vi "Detect Framework From Application Domain.vi"(8 "error in (no error)":errorcluster) -> (0 "error out":errorcluster, 1 "Test Framework Instance":refnum<class "Test Framework.lvclass">, 2 "Test Framework Type":T1=enum."LVUnit")   [LabVIEW 2017, in "Framework.lvlib" / "Test Framework Factory.lvclass"]
uses:
  Test Framework Factory.lvclass
  Test Framework/Test Framework.lvclass
  Test Framework.ctl
  LVUnit Test Framework/LVUnit Test Framework.lvclass
  C:/Users/pasca/Projects/Home/lvunit/Framework/Test Framework/Test Framework.lvclass
  Framework.lvlib
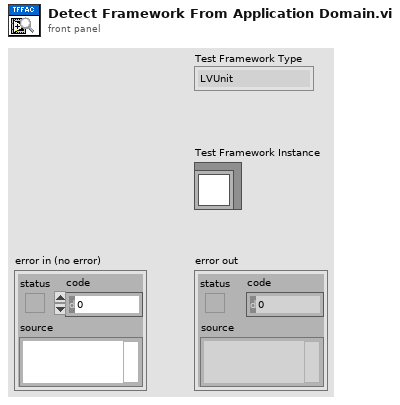
[diagram p1: front panel]
types:
  T1 = typedef "Framework.lvlib/Test Framework.ctl" = enum16{"Unknown", "LVUnit"}
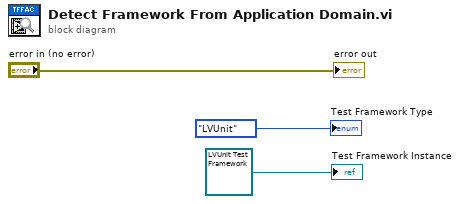
[diagram p0: block diagram]
diagram:
  "error out" <- "error in (no error)"
  "Test Framework Instance" <- refnum<class "LVUnit Test Framework.lvclass"> refnum ("Framework.lvlib:LVUnit Test Framework.lvclass")
  "Test Framework Type" <- Test_Framework."LVUnit" ("Test Framework")
